vi "Begin.vi"(8 "error in":errorcluster) -> (0 "error out":errorcluster)   [LabVIEW 2017]
doc: "Called before other user functions, this VI is expected to open initial I/O refnums, load in file data, and do all program initialization. Notice that the <B>error out</B> terminal is simply used for data flow. Wiring it to other structures or subVIs ensures that this VI runs first."
uses:
  <vilib>/Rock Robotics/WPI/Joystick/WPI_JoystickDeviceEnum.ctl
  <vilib>/Rock Robotics/WPI/DriverStation/WPI_DriverStationRobotMode2.ctl
  <vilib>/Rock Robotics/SystemInterfaces/DIO/FPGA_DIOPWMChannel.ctl
  <vilib>/Rock Robotics/WPI/SafetyOutput/WPI_SafetyOutputConfigMenu.ctl
  <vilib>/Rock Robotics/SystemInterfaces/spilib/spi_bus.ctl
  <vilib>/Rock Robotics/Network Tables/NT Write String Array.vi
  Robot Global Data.vi
  Global Variables.vi
  <vilib>/Rock Robotics/WPI/RobotDrive/WPI_RobotDriveOpen4MotorWithSPARK.vi
  <vilib>/Rock Robotics/WPI/RobotDrive/WPI_RobotDriveOpen2MotorWithSPARK.vi
  <vilib>/Rock Robotics/WPI/RobotDrive/WPI_RobotDriveOpen2MotorWithVictor.vi
  <vilib>/Rock Robotics/WPI/Gyro/WPI_GyroXRS450_SPI_Open.vi
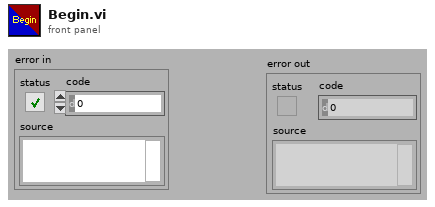
[diagram p1: front panel]
types:
  T1 = typedef "WPI_DriverStationRobotMode2.ctl" = enum16{"Autonomous Disabled", "Autonomous Enabled", "Teleop Disabled", "Teleop Enabled", "Disconnected", "Finish", "Test Disabled", "Test Enabled", "Emergency Stopped"}
  T2 = typedef "WPI_JoystickDeviceEnum.ctl" = enum16{"USB 0", "USB 1", "USB 2", "USB 3", "USB 4", "USB 5"}
  T3 = typedef "WPI_SafetyOutputConfigMenu.ctl" = enum16{"Enable", "Disable"}
  T4 = typedef "spi_bus.ctl" = enum16{"SPI On-Board, CS0", "SPI On-Board, CS1", "SPI On-Board, CS2", "SPI On-Board, CS3", "SPI MXP", "Invalid"}
  T5 = typedef "WPI_JoystickDevRef.ctl" = cluster{"Device":T2}
  T6 = typedef "FPGA_DIOPWMChannel.ctl" = enum8{"PWM 0", "PWM 1", "PWM 2", "PWM 3", "PWM 4", "PWM 5", "PWM 6", "PWM 7", "PWM 8", "PWM 9", "PWM MXP 0", "PWM MXP 1", "PWM MXP 2", "PWM MXP 3", "PWM MXP 4", "PWM MXP 5", "PWM MXP 6", "PWM MXP 7", "PWM MXP 8", "PWM MXP 9", "Invalid"}
  T7 = typedef "WPI_RobotDriveDevRef.ctl" = cluster{"DevStatus":errorcluster, "Motors[]":T8[], "Square Inputs":bool, "Max Output":dbl}
  T8 = typedef "WPI_MotorControlDeviceRef.ctl" = cluster{"DeviceStatus":errorcluster, "Type":T9, "PWM":cluster{"PWM Channel":T6, "DeadBand":T10}, "CAN":cluster{"Device Number":u8, "SetOutput VI Ref":variant, "GetOutput VI Ref":variant, "Enable VI Ref":variant, "Disable VI Ref":variant, "Data":variant}, "Invert":bool, "DIO PWM":cluster{"PWM \"Enable\" Channel":T6, "DIOChannel":T11, "PWM Rate":dbl}}
  T9 = typedef "WPI_MotorControlType.ctl" = enum16{"PWM", "CAN", "DIO PWM"}
  T10 = typedef "WPI_PWMDeadband.ctl" = cluster{"Name":string, "maxPositivePwm":i32, "minPositivePwm":i32, "centerPwm":i32, "maxNegativePwm":i32, "minNegativePwm":i32, "angularRange":u16}
  T11 = typedef "FPGA_DIOChannel.ctl" = enum8{"DIO 0", "DIO 1", "DIO 2", "DIO 3", "DIO 4", "DIO 5", "DIO 6", "DIO 7", "DIO 8", "DIO 9", "DIO MXP 0", "DIO MXP 1", "DIO MXP 2", "DIO MXP 3", "DIO MXP 4", "DIO MXP 5", "DIO MXP 6", "DIO MXP 7", "DIO MXP 8", "DIO MXP 9", "DIO MXP 10", "DIO MXP 11", "DIO MXP 12", "DIO MXP 13", "DIO MXP 14", "DIO MXP 15", "SPI Port CS1", "SPI Port CS2", "SPI Port CS3", "SPI Port MISO", "SPI Port MOSI", "Invalid"}
  T12 = typedef "WPI_GyroDevRef.ctl" = cluster{"DevStatus":errorcluster, "Analog Channel":T13, "Gain (VoltsPerDegree/Second)":dbl, "Gyro Type":enum16{"Analog", "XRS450"}, "Handle":i32, "SPI Bus":T4, "Device Found":bool, "Sample Rate":dbl, "Calibrate On Open":bool, "Offset":dbl}
  T13 = typedef "FPGA_AIChannel.ctl" = enum8{"AI 0", "AI 1", "AI 2", "AI 3", "AI MXP 0", "AI MXP 1", "AI MXP 2", "AI MXP 3", "Invalid"}
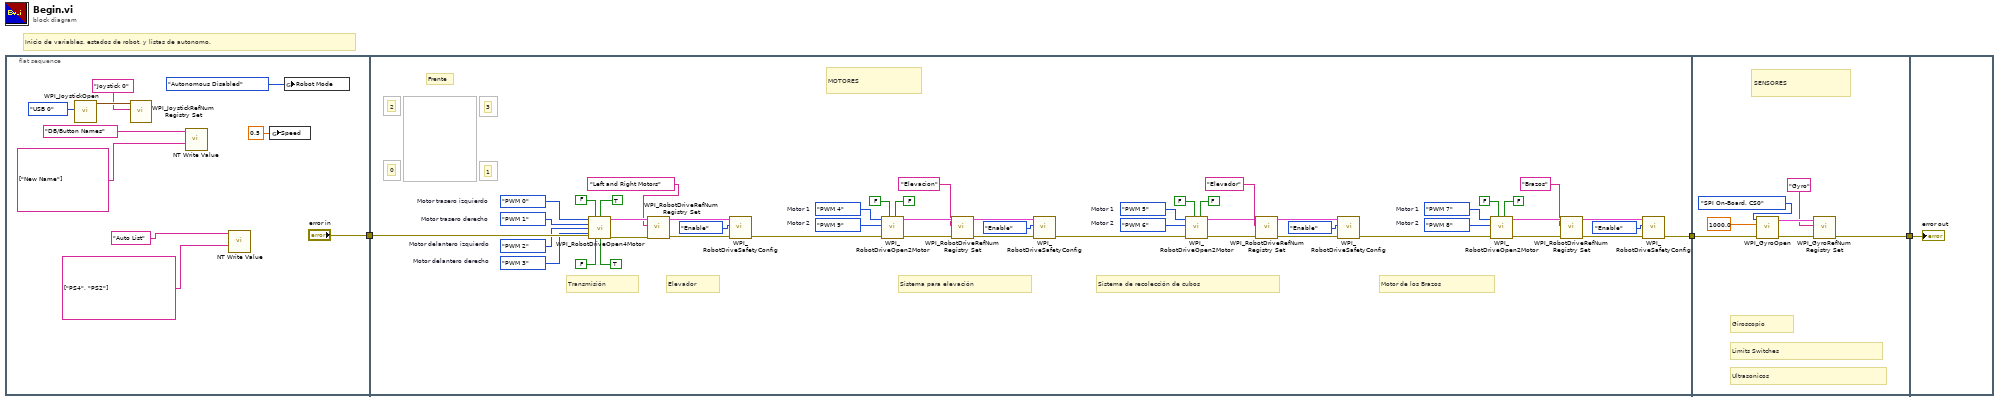
[diagram p0: block diagram]
diagram:
  # "Inicio de variables, estados de robot, y listas de autonomo."
  n1 = flat-sequence {
    tunnel: ["error in"] -> w3
    tunnel: w3 -> [w52]
    tunnel: [w26] -> w2
    tunnel: w2 -> [w69]
    tunnel: [w63] -> w1
    tunnel: w1 -> [w70]
    frame #0 {
      n2 = call <vilib>:"WPI_JoystickOpen.vi"("JoystickDevice"=WPI_JoystickDeviceEnum."USB 0") -> ("JoystickDevRef"=w12:T5)  [unwired: 10 in]
      n3 = call <vilib>:"WPI_JoystickRefNum Registry Set.vi"("refnum name"="Joystick 0", "JoystickDevRef"=w12) -> ()  [unwired: 8 in, 2 out]
      n4 = call-poly <vilib>:"NT Write Value.vi"("String Array"=string[] ["New Name"], "Name"="DB/Button Names") -> ()  [unwired: 9 in, 1 out]
      n5 = call-poly <vilib>:"NT Write Value.vi"("String Array"=string[] ["PS4", "PS2"], "Name"="Auto List") -> ()  [unwired: 9 in, 1 out]
      n6 = global write "Global Variables.vi" "Speed"(0.5 ("Speed")) -> ()
      n7 = global write "Robot Global Data.vi" "Robot Mode"(WPI_DriverStationRobotMode2."Autonomous Disabled" ("Robot Mode")) -> ()
    }
    frame #1 {
      w16 = FPGA_DIOPWMChannel."PWM 9"  # Motor 2
      w17 = FPGA_DIOPWMChannel."PWM 4"  # Motor 1
      w37 = FPGA_DIOPWMChannel."PWM 6"  # Motor 2
      w36 = FPGA_DIOPWMChannel."PWM 5"  # Motor 1
      w38 = FPGA_DIOPWMChannel."PWM 8"  # Motor 2
      w39 = FPGA_DIOPWMChannel."PWM 7"  # Motor 1
      w48 = FPGA_DIOPWMChannel."PWM 3"  # Motor delantero derecho
      w49 = FPGA_DIOPWMChannel."PWM 2"  # Motor delantero izquierdo
      w50 = FPGA_DIOPWMChannel."PWM 1"  # Motor trasero derecho
      w51 = FPGA_DIOPWMChannel."PWM 0"  # Motor trasero izquierdo
      # "Sistema para elevación"
      # "Motor de los Brazos"
      # "Sistema de recolección de cubos"
      # "Elevador"
      # "Transmisión"
      # "MOTORES"
      # "Frente"
      # "0"
      # "2"
      # "1"
      # "3"
      n8 = call-poly <vilib>:"WPI_RobotDriveOpen4Motor.vi"("Rear Left Motor"=w51, "Rear Left Motor Inverted"=FALSE, "Rear Right Motor Inverted"=TRUE, "Rear Right Motor"=w50, "Front Left Motor"=w49, "Front Right Motor"=w48, "error in (no error)"=w52, "Front Left Motor Inverted"=FALSE ("Rear Left Motor Inverted"), "Front Right Motor Inverted"=TRUE ("Rear Right Motor Inverted")) -> ("RobotDriveDevRef"=w61:T7, "error out"=w55:errorcluster)  [unwired: 5 in]
      n9 = call <vilib>:"WPI_RobotDriveRefNum Registry Set.vi"("error in (no error)"=w55, "refnum name"="Left and Right Motors", "RobotDriveDevRef"=w61) -> ("error out"=w56:errorcluster, "RobotDriveDevRef"=w62:T7)  [unwired: 1 in, 6 out]
      n10 = call <vilib>:"WPI_RobotDriveSafetyConfig.vi"("error in (no error)"=w56, "mode"=WPI_SafetyOutputConfigMenu."Enable", "RobotDriveDevRef"=w62) -> ("error out"=w15:errorcluster)  [unwired: 7 in, 1 out]
      n11 = call-poly <vilib>:"WPI_RobotDriveOpen2Motor.vi"("Right Motor Inverted"=FALSE, "Left Motor Inverted"=FALSE, "error in (no error)"=w15, "Right Motor"=w16, "Left Motor"=w17) -> ("error out"=w24:errorcluster, "RobotDriveDevRef"=w25:T7)  [unwired: 5 in]
      n12 = call <vilib>:"WPI_RobotDriveRefNum Registry Set.vi"("error in (no error)"=w24, "refnum name"="Elevacion", "RobotDriveDevRef"=w25) -> ("error out"=w23:errorcluster, "RobotDriveDevRef"=w22:T7)  [unwired: 7 in]
      n13 = call <vilib>:"WPI_RobotDriveSafetyConfig.vi"("error in (no error)"=w23, "mode"=WPI_SafetyOutputConfigMenu."Enable", "RobotDriveDevRef"=w22) -> ("error out"=w14:errorcluster)  [unwired: 7 in, 1 out]
      n14 = call-poly <vilib>:"WPI_RobotDriveOpen2Motor.vi"("Right Motor Inverted"=FALSE, "Left Motor Inverted"=FALSE, "error in (no error)"=w14, "Right Motor"=w37, "Left Motor"=w36) -> ("error out"=w29:errorcluster, "RobotDriveDevRef"=w28:T7)  [unwired: 5 in]
      n15 = call <vilib>:"WPI_RobotDriveRefNum Registry Set.vi"("error in (no error)"=w29, "refnum name"="Elevador", "RobotDriveDevRef"=w28) -> ("error out"=w30:errorcluster, "RobotDriveDevRef"=w31:T7)  [unwired: 7 in]
      n16 = call <vilib>:"WPI_RobotDriveSafetyConfig.vi"("error in (no error)"=w30, "mode"=WPI_SafetyOutputConfigMenu."Enable", "RobotDriveDevRef"=w31) -> ("error out"=w27:errorcluster)  [unwired: 7 in, 1 out]
      n17 = call-poly <vilib>:"WPI_RobotDriveOpen2Motor.vi"("Right Motor Inverted"=FALSE, "Left Motor Inverted"=FALSE, "error in (no error)"=w27, "Right Motor"=w38, "Left Motor"=w39) -> ("error out"=w46:errorcluster, "RobotDriveDevRef"=w47:T7)  [unwired: 5 in]
      n18 = call <vilib>:"WPI_RobotDriveRefNum Registry Set.vi"("error in (no error)"=w46, "refnum name"="Brazos", "RobotDriveDevRef"=w47) -> ("error out"=w45:errorcluster, "RobotDriveDevRef"=w44:T7)  [unwired: 7 in]
      n19 = call <vilib>:"WPI_RobotDriveSafetyConfig.vi"("error in (no error)"=w45, "mode"=WPI_SafetyOutputConfigMenu."Enable", "RobotDriveDevRef"=w44) -> ("error out"=w26:errorcluster)  [unwired: 7 in, 1 out]
    }
    frame #2 {
      # "Ultrasonicos"
      # "Limits Switches"
      # "Giroscopio"
      # "SENSORES"
      n20 = call-poly <vilib>:"WPI_GyroOpen.vi"("error in"=w69, "Sample Rate (Hz)"=1000.0, "SPI Bus"=spi_bus."SPI On-Board, CS0") -> ("error out"=w67:errorcluster, "GyroDevRef"=w68:T12)  [unwired: 6 in, 1 out]
      n21 = call <vilib>:"WPI_GyroRefNum Registry Set.vi"("error in (no error)"=w67, "refnum name"="Gyro", "GyroDevRef"=w68) -> ("error out"=w63:errorcluster)  [unwired: 7 in, 1 out]
    }
    frame #3 {
      "error out" <- w70
    }
  }
